vi "SetOutputVoltage.vi"(8 "error in (no error)":errorcluster, 10 "Voltage":dbl, 11 "RMX4120 in":refnum<class "RMX4120.lvclass">) -> (0 "error out":errorcluster, 3 "RMX4120 out":refnum<class "RMX4120.lvclass">)   [LabVIEW 2023, in "RMX4120.lvclass"]
uses:
  RMX4120.lvclass
  RMX4120.lvclass/RMX4120.ctl
  RMXPowerSupply.lvclass
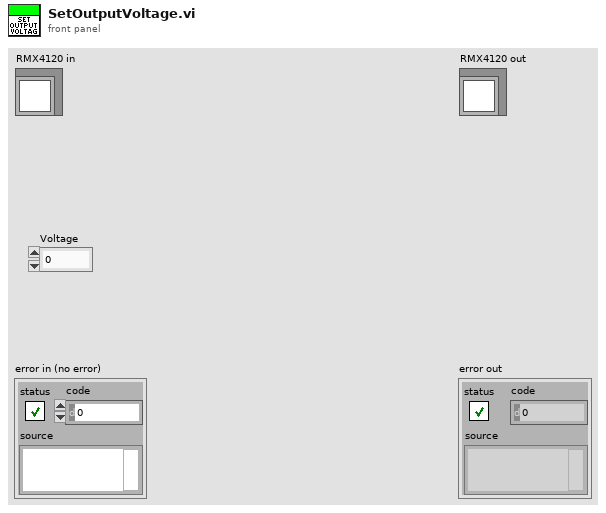
[diagram p1: front panel]
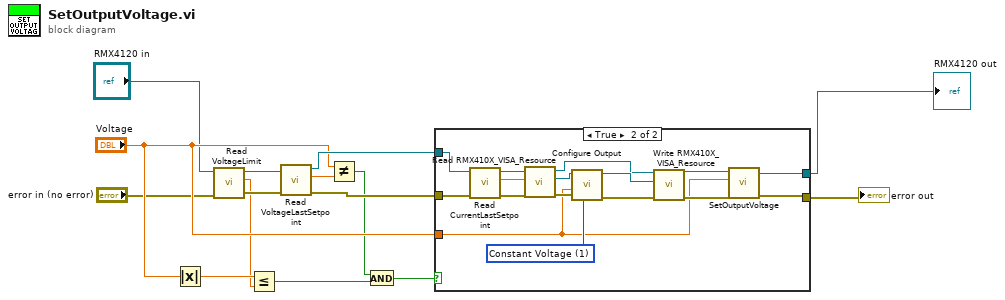
[diagram p0: block diagram]
diagram:
  n1 = Absolute Value(x="Voltage") -> (abs(x)=w10:dbl)
  n2 = call-dynamic "Read VoltageLimit.vi"("error in (no error)"="error in (no error)", "RMXPowerSupply in"="RMX4120 in") -> ("error out"=w5:errorcluster, "VoltageLimit"=w3:dbl, "RMXPowerSupply out"=w7:refnum<class "RMX4120.lvclass">)  [unwired: 7 in]
  n3 = Less Or Equal?(x=w10, y=w3) -> (x <= y?=w9:bool)
  n4 = call-dynamic "Read VoltageLastSetpoint.vi"("error in (no error)"=w5, "RMXPowerSupply in"=w7) -> ("error out"=w13:errorcluster, "VoltageLastSetpoint"=w15:dbl, "RMXPowerSupply out"=w14:refnum<class "RMX4120.lvclass">)  [unwired: 7 in]
  n5 = Not Equal?(x="Voltage", y=w15) -> (x != y?=w2:bool)
  n6 = And(x=w2, y=w9) -> (x .and. y?=w1:bool)
  n7 = case shown="True" w1 {
    tunnel: w14 -> [w17 w28]
    tunnel: w13 -> [w16 w30]
    tunnel: "Voltage" -> [_ w18]
    tunnel: [w17 w20] -> w12
    tunnel: [w16 w21] -> w11
    frame False {
    }
    frame True {
      w31 = 1 items=["Constant Current", "Constant Voltage"] ("Operation Mode (0: Constant Current)")
      n8 = call-dynamic "Read CurrentLastSetpoint.vi"("error in (no error)"=w30, "RMXPowerSupply in"=w28) -> ("error out"=w29:errorcluster, "CurrentLastSetpoint"=w26:dbl, "RMXPowerSupply out"=w27:refnum<class "RMX4120.lvclass">)  [unwired: 7 in]
      n9 = call-dynamic "Read RMX410X_VISA_Resource.vi"("error in (no error)"=w29, "RMXPowerSupply in"=w27) -> ("error out"=w32:errorcluster, "RMX410X_VISA_Resource"=w33:refnum<visa-resource-name>, "RMXPowerSupply out"=w24:refnum<class "RMX4120.lvclass">)  [unwired: 7 in]
      n10 = call "Configure Output.vi"("Operation Mode (0: Constant Current)"=w31, "error in (no error)"=w32, "Output Voltage (0 V)"=w18, "Output Current (0 A)"=w26, "VISA resource name"=w33) -> ("error out"=w23:errorcluster, "VISA resource name out"=w25:refnum<visa-resource-name>)  [unwired: 5 in]
      n11 = call-dynamic "Write RMX410X_VISA_Resource.vi"("error in (no error)"=w23, "RMX410X_VISA_Resource"=w25, "RMXPowerSupply in"=w24) -> ("error out"=w22:errorcluster, "RMXPowerSupply out"=w19:refnum<class "RMX4120.lvclass">)  [unwired: 7 in]
      n12 = call-parent "SetOutputVoltage.vi"("error in (no error)"=w22, "Voltage"=w18, "RMXPowerSupply in"=w19) -> ("error out"=w21:errorcluster, "RMXPowerSupply out"=w20:refnum<class "RMX4120.lvclass">)  [unwired: 7 in]
    }
  }
  "error out" <- w11
  "RMX4120 out" <- w12
